vi "Cube Drop.vi"   [LabVIEW 2020, in "VolatusDAQGenericGUI.lvlib"]
uses:
  VolatusDAQGenericGUI.lvlib
  GenericGuiDO/GenericGuiDO.lvclass
  GenericGuiDI/GenericGuiDI.lvclass
  GenericGuiAO/GenericGuiAO.lvclass
  GenericGuiAI/GenericGuiAI.lvclass
  VolatusGUI/VolatusGUI.lvlib
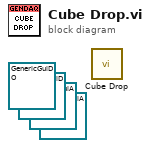
[diagram p0: block diagram]
diagram:
  (unwired) refnum<class "GenericGuiAI.lvclass"> refnum ("VolatusDAQGenericGUI.lvlib:GenericGuiAI.lvclass")
  (unwired) refnum<class "GenericGuiAO.lvclass"> refnum ("VolatusDAQGenericGUI.lvlib:GenericGuiAO.lvclass")
  (unwired) refnum<class "GenericGuiDI.lvclass"> refnum ("VolatusDAQGenericGUI.lvlib:GenericGuiDI.lvclass")
  (unwired) refnum<class "GenericGuiDO.lvclass"> refnum ("VolatusDAQGenericGUI.lvlib:GenericGuiDO.lvclass")
  n1 = call "Cube Drop.vi"() -> ()  [unwired: 12 in]
